vi "EON_pres_abs_threshold.vi"(8 "error in (no error)":errorcluster, 10 "ROI Descriptor":T1 {"Contours"."Type" items=["No Selection", "Point", "Line", "Rectangle", "Oval", "Polygon", "Freehand Region", "Annulus", "Unused2", "Unused3", "Broken Line", "Freehand Line", "Rotated Rectangle"]}, 11 "Image In":T2(plugin-control)) -> (0 "error out":errorcluster, 3 "EON Present?":dbl)   [LabVIEW 2015]
uses:
  <vilib>/vision/NI_Vision_Development_Module.lvlib
panel:
  out "x > y?":bool
  out "Image Dst Out":T2(plugin-control)
  out "Area":dbl
  out "subarray":dbl[](array[numeric])
  out "Array":bool[](array[boolean])
  out "Binary Image":T2(plugin-control)
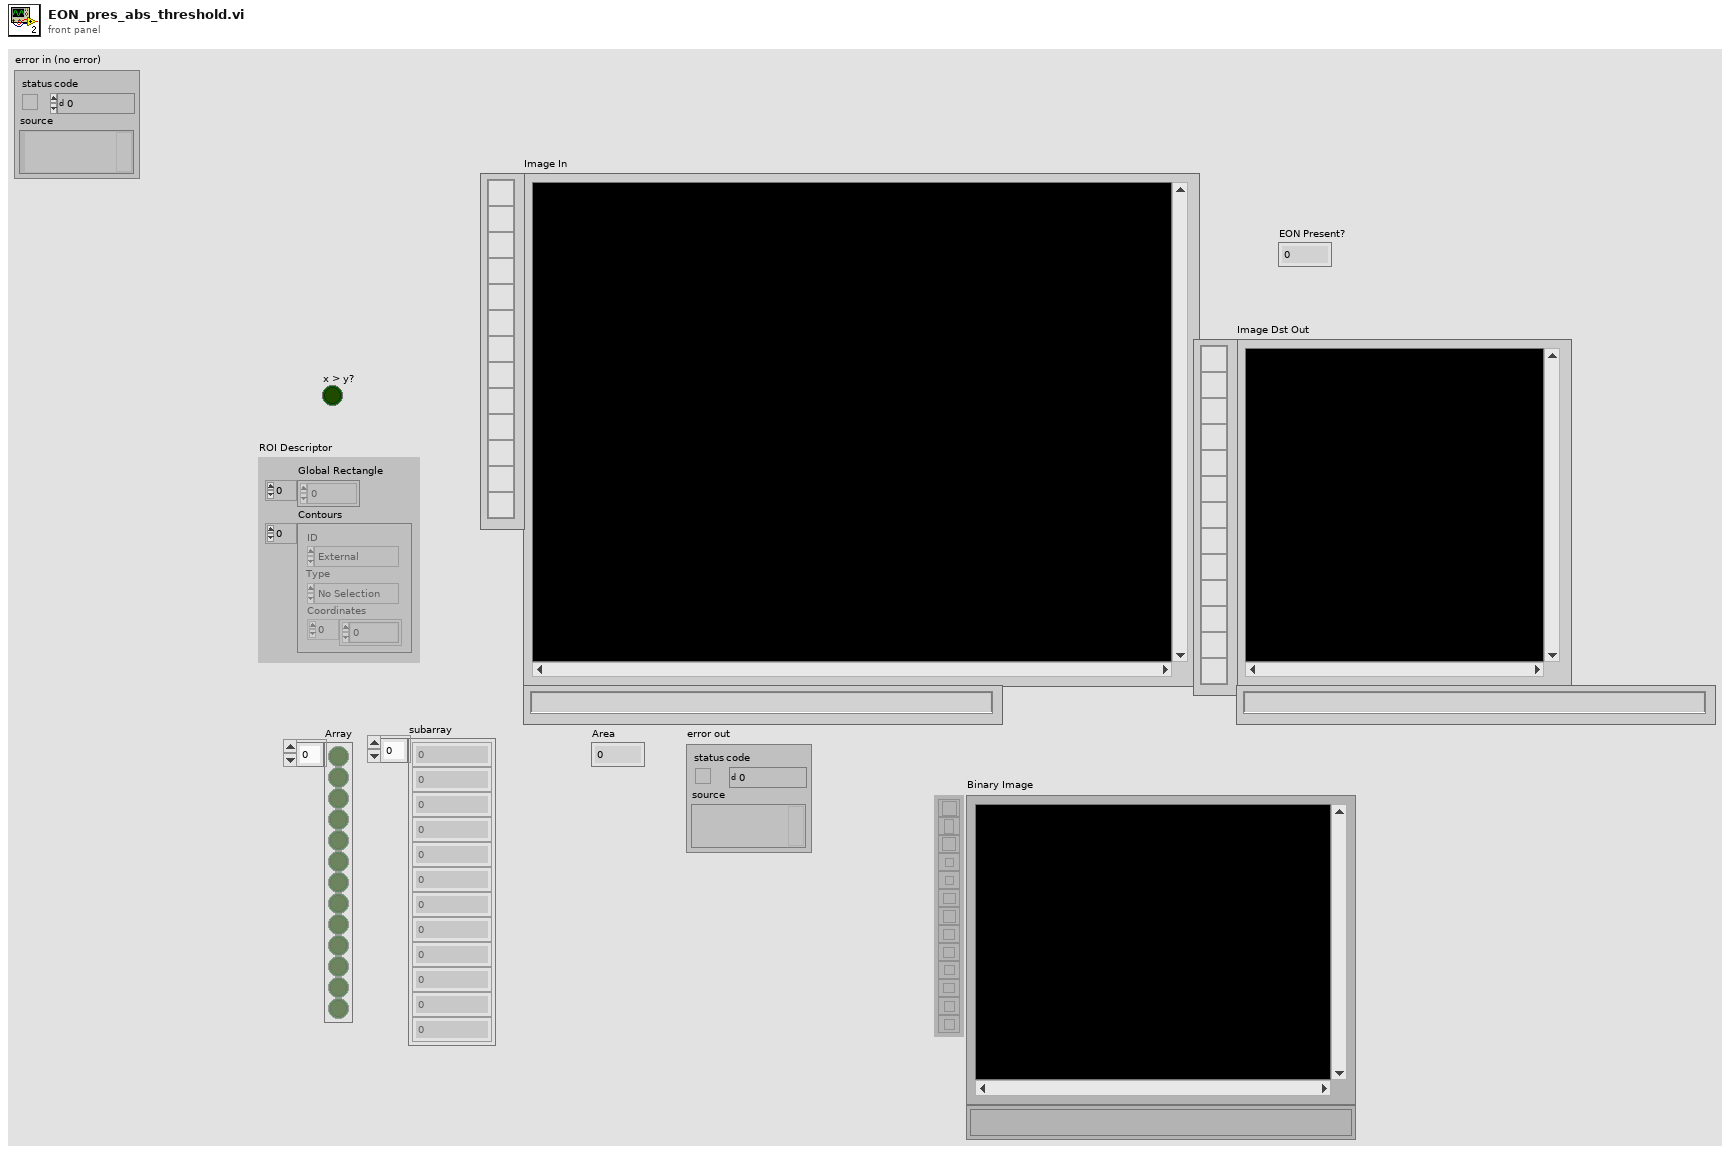
[diagram p1: front panel]
types:
  T1 = typedef "ROI Descriptor" = cluster{"Global Rectangle":i32[], "Contours":cluster{"ID":enum32{"External", "Internal"}, "Type":u32, "Coordinates":i32[]}[]}
  T2 = typedef "IMAQ Image.ctl" = refnum<image>
  T3 = cluster{"Origin":cluster{"X":sgl, "Y":sgl}, "Angle (deg)":sgl, "Axis Reference":u32}
  T4 = typedef "Particle Parameters" = i32
  T5 = cluster{"Measurement Parameter":T4, "Range Lower Value":dbl, "Range Upper Value":dbl, "Range":bool, "Measurement Type":bool}[]
  T6 = typedef "IMAQ Rectangle" = cluster{"Left":i32, "Top":i32, "Right":i32, "Bottom":i32, "Rotation":dbl}
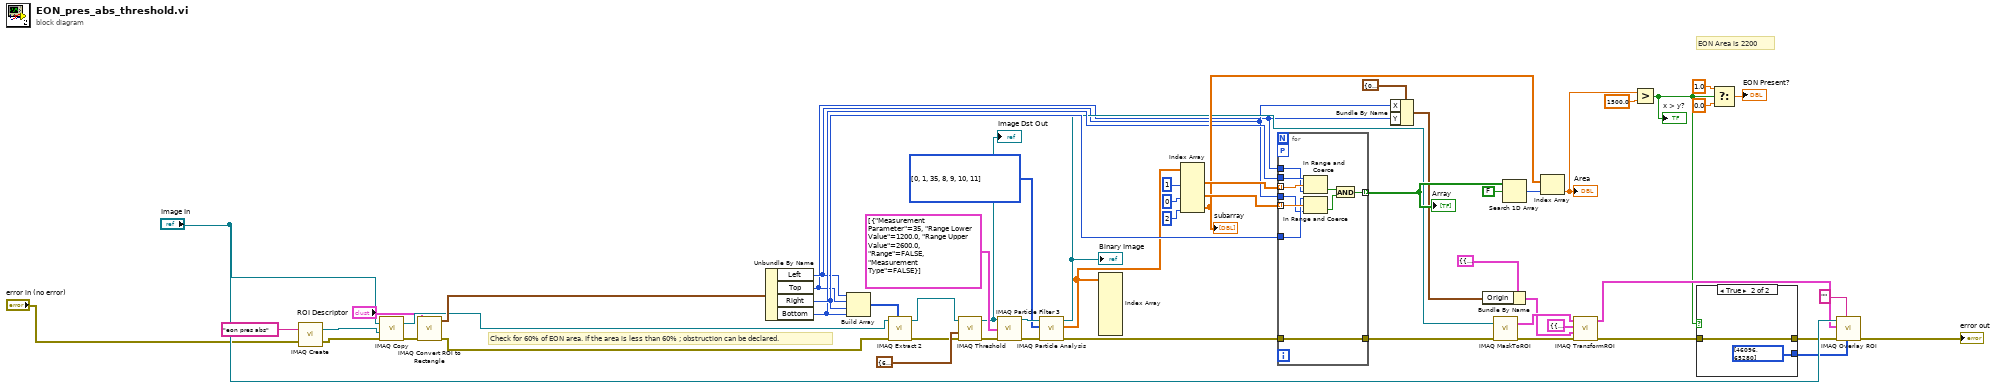
[diagram p0: block diagram]
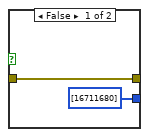
[diagram p2: hidden frame]
diagram:
  w48 = T4[] [0, 1, 35, 8, 9, 10, 11] items=["Center of Mass X", "Center of Mass Y", "First Pixel X", "First Pixel Y", "Bounding Rect Left", "Bounding Rect Top", "Bounding Rect Right", "Bounding Rect Bottom", "Max Feret Diameter Start X", "Max Feret Diameter Start Y", "Max Feret Diameter End X", "Max Feret Diameter End Y", "Max Horiz. Segment Length Left", "Max Horiz. Segment Length Right", "Max Horiz. Segment Length Row", "-", "Bounding Rect Width", "Bounding Rect Height", "Bounding Rect Diagonal", "Perimeter", "Convex Hull Perimeter", "Holes' Perimeter", "Max Feret Diameter", "Equivalent Ellipse Major Axis", "Equivalent Ellipse Minor Axis", "Equivalent Ellipse Minor Axis (Feret)", "Equivalent Rect Long Side", "Equivalent Rect Short Side", "Equivalent Rect Diagonal", "Equivalent Rect Short Side (Feret)", "Average Horiz. Segment Length", "Average Vert. Segment Length", "Hydraulic Radius", "Waddel Disk Diameter", "-", "Area", "Holes' Area", "Particle & Holes' Area", "Convex Hull Area", "Image Area", "-", "Number of Holes", "Number of Horiz. Segments", "Number of Vert. Segments", "-", "Orientation", "Max Feret Diameter Orientation", "-", "% Area/Image Area", "% Area/(Particle & Holes' Area)", "Ratio of Equivalent Ellipse Axes", "Ratio of Equivalent Rect Sides", "-", "Elongation Factor", "Compactness Factor", "Heywood Circularity Factor", "Type Factor", "-", "Sum X", "Sum Y", "Sum XX", "Sum XY", "Sum YY", "Sum XXX", "Sum XXY", "Sum XYY", "Sum YYY", "-", "Moment of Inertia XX", "Moment of Inertia XY", "Moment of Inertia YY", "Moment of Inertia XXX", "Moment of Inertia XXY", "Moment of Inertia XYY", "Moment of Inertia YYY", "Norm. Moment of Inertia XX", "Norm. Moment of Inertia XY", "Norm. Moment of Inertia YY", "Norm. Moment of Inertia XXX", "Norm. Moment of Inertia XXY", "Norm. Moment of Inertia XYY", "Norm. Moment of Inertia YYY", "Hu Moment 1", "Hu Moment 2", "Hu Moment 3", "Hu Moment 4", "Hu Moment 5", "Hu Moment 6", "Hu Moment 7"] ("Pixel Measurements")
  # "EON Area is 2200"
  # "Check for 60% of EON area. If the area is less than 60% ; obstruction can be declared."
  n1 = call "IMAQ Create"("Image Name"="eon pres abs", "error in (no error)"="error in (no error)") -> ("New Image"=w29:T2, "error out"=w31:errorcluster)  [unwired: 3 in]
  n2 = call "IMAQ Copy"("error in (no error)"=w31, "Image Dst"=w29, "Image Src"="Image In") -> ("error out"=w27:errorcluster, "Image Dst Out"=w21:T2)  [unwired: 3 in]
  n3 = call "IMAQ Convert ROI to Rectangle"("error in (no error)"=w27, "ROI Descriptor"="ROI Descriptor") -> ("error out"=w26:errorcluster, "Rectangle"=w22:T6)  [unwired: 7 in]
  n4 = Unbundle By Name(w22) -> ("Left"=w10:i32, "Top"=w9:i32, "Right"=w34:i32, "Bottom"=w28:i32)
  n5 = Build Array(w10, w9, w34, w28) -> (w33:i32[])
  n6 = call "IMAQ Extract 2"("Optional Rectangle"=w33, "error in (no error)"=w26, "Image Src"=w21) -> ("error out"=w36:errorcluster, "Image Dst Out"=w32:T2)  [unwired: 7 in]
  n7 = call "IMAQ Threshold"("error in (no error)"=w36, "Range"=cluster{"Lower value":sgl, "Upper value":sgl} {"Lower value"=60.0, "Upper value"=255.0}, "Image Src"=w32) -> ("error out"=w51:errorcluster, "Image Dst Out"=w50:T2)  [unwired: 7 in]
  "Image Dst Out" <- w50
  n8 = call "IMAQ Particle Filter 3"("Image Src"=w50, "Selection Values"=T5 [{"Measurement Parameter"=35, "Range Lower Value"=1200.0, "Range Upper Value"=2600.0, "Range"=FALSE, "Measurement Type"=FALSE}], "error in (no error)"=w51) -> ("Image Dst Out"=w53:T2, "error out"=w54:errorcluster)  [unwired: 10 in, 1 out]
  n9 = call "IMAQ Particle Analysis"("error in (no error)"=w54, "Pixel Measurements"=w48, "Image"=w53) -> ("error out"=w35:errorcluster, "Particle Measurements (Pixels)"=w20:dbl[][], "Image Out (duplicate)"=w19:T2)  [unwired: 3 in, 3 out]
  "Binary Image" <- w19
  n10 = Index Array(array=w20) -> ()  [unwired: 8 in, 4 out]
  n11 = Index Array(array=w20, index (col) #1=1 ("disabled index (col)"), index (col) #2=0 ("index (col)"), index (col) #3=2 ("index (col)")) -> (element #1=w46:dbl[], element #2=w44:dbl[], element #3=w40:dbl[])  [unwired: 3 in]
  "subarray" <- w40
  n12 = for {
    tunnel: w46 -> [w66] mode=indexing
    tunnel: [w61] -> w42 mode=indexing
    tunnel: w28 -> [w65]
    tunnel: w9 -> [w64]
    tunnel: w44 -> [w62] mode=indexing
    tunnel: w34 -> [w59]
    tunnel: w10 -> [w58]
    tunnel: w35 -> [w57]
    tunnel: [w57] -> w8
    workers-P: _ -> [_]
    n13 = In Range and Coerce(upper limit=w65, x=w66, lower limit=w64) -> (In Range?=w63:bool)  [unwired: 1 out]
    n14 = In Range and Coerce(upper limit=w59, x=w62, lower limit=w58) -> (In Range?=w60:bool)  [unwired: 1 out]
    n15 = And(x=w63, y=w60) -> (x .and. y?=w61:bool)
  }
  "Array" <- w42
  n16 = Bundle By Name(cluster=cluster{"X":sgl, "Y":sgl} {"X"=0.0, "Y"=0.0} ("Origin"), "X"=w10, "Y"=w9) -> (w12:cluster{"X":sgl, "Y":sgl})
  n17 = Bundle By Name(cluster=T3 {"Origin"={"X"=0.0, "Y"=0.0}, "Angle (deg)"=0.0, "Axis Reference"=0} ("Base Reference"), "Origin"=w12) -> (w11:T3)
  n18 = call "IMAQ MaskToROI"("Image"=w19, "error in (no error)"=w8) -> ("ROI Descriptor"=w18:T1, "error out"=w7:errorcluster)  [unwired: 5 in, 1 out]
  n19 = Search 1D Array(1D array=w42, element=FALSE) -> (index of element=w39:i32)  [unwired: 1 in]
  n20 = Index Array(array=w40, index=w39) -> (element=w38:dbl)
  "Area" <- w38
  n21 = call "IMAQ TransformROI"("error in (no error)"=w7, "New Reference"=w11, "Base Reference"=T3 {"Origin"={"X"=0.0, "Y"=0.0}, "Angle (deg)"=0.0, "Axis Reference"=0}, "ROI Descriptor"=w18) -> ("error out"=w5:errorcluster, "ROI Descriptor out"=w15:T1)  [unwired: 6 in]
  n22 = Greater?(x=w38, y=1500.0) -> (0:w6:bool)
  "x > y?" <- w6
  n23 = case shown="True" w6 {
    tunnel: [u32[] [16711680] ("Colors (Green)") u32[] [46096, 65280] ("Colors (Green)")] -> w17
    tunnel: w5 -> [w67 w69]
    tunnel: [w67 w69] -> w4
    frame False {
    }
    frame True {
    }
  }
  n24 = Select(t=1.0, s=w6, f=0.0) -> (s? t:f=→"EON Present?":dbl)
  n25 = call "IMAQ Overlay ROI"("Colors (Green)"=w17, "Group"="", "error in (no error)"=w4, "ROI Descriptor"=w15, "Image"="Image In") -> ("error out"=→"error out":errorcluster)  [unwired: 5 in, 1 out]
